vi "Initialize Transfer Groups.vi"(7 "FIFO Options":T1, 8 "error in (no error)":errorcluster, 10 "Transfer Group configurations":T2[](array[typedef]) {"Transfers"."channel blocks"."string descriptor"."buffer offset" format="%d bytes"; "Transfers"."channel blocks"."engine descriptor"."buffer offset" format="%d bytes"}, 11 "Plugin in":refnum<class "Plugin.lvclass">) -> (0 "error out":errorcluster, 2 "Transfer Groups":refnum<class "Transfer Group.lvclass">[](array[class]), 3 "Plugin out":refnum<class "Plugin.lvclass">)   [LabVIEW 2017, in "DSF Core.lvlib" / "Plugin.lvclass"]
uses:
  Plugin.lvclass
  DSF Configuration API/Public/Controls/DSF Engine Transfer Group Configuration.ctl
  DSF Configuration API/Public/Controls/DSF Direction.ctl
  DSF Configuration API/Public/Controls/DSF Timing Info.ctl
  DSF Configuration API/Public/Controls/DSF Settings Info.ctl
  DSF Configuration API/Public/Controls/DSF Engine Transfer Configuration.ctl
  DSF Configuration API/Public/Controls/DSF Byte Order.ctl
  DSF Configuration API/Public/Controls/DSF Engine Channel Configuration.ctl
  DSF Configuration API/Public/Controls/DSF Channel Buffer Descriptor.ctl
  DSF Configuration API/Public/Controls/DSF Data Type.ctl
  Transfer Group/Transfer Group.lvclass
  Typedefs/FIFO Flags.ctl
  Plugin.lvclass/Plugin.ctl
  Transfer Group/Transfer Group.lvclass/Transfer Group.ctl
  Shared/VIs/Sizeof.vi
  DSF Configuration API/Public/Required Buffer Size (Transfer Group).vi
  DSF Configuration API/Public/Channel Count (Transfer Group).vi
  DSF Core.lvlib
  Buffer/Buffers.lvclass
  Timing/Timing.lvclass
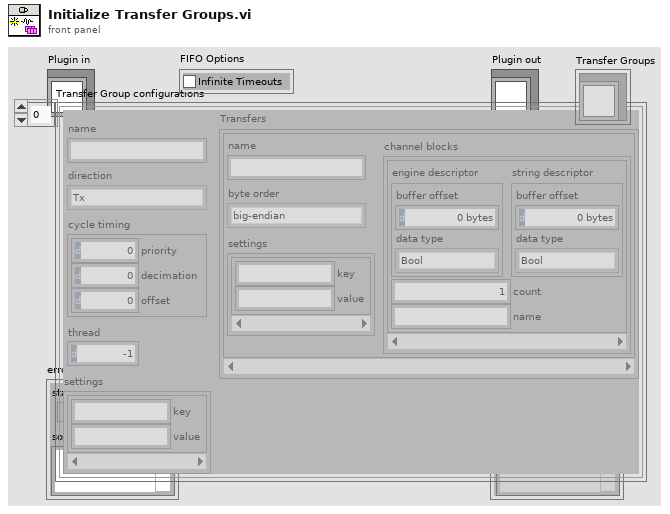
[diagram p1: front panel]
types:
  T1 = typedef "DSF Core.lvlib/FIFO Flags.ctl" = cluster{"Infinite Timeouts":bool}
  T2 = typedef "DSF Core.lvlib/DSF Engine Transfer Group Configuration.ctl" = cluster{"name":string, "direction":T3, "cycle timing":T4, "thread":i32, "settings":T5, "Transfers":T6[]}
  T3 = typedef "DSF Core.lvlib/DSF Direction.ctl" = enum8{"Tx", "Rx"}
  T4 = typedef "DSF Core.lvlib/DSF Timing Info.ctl" = cluster{"priority":u64, "decimation":u64, "offset":u64}
  T5 = typedef "DSF Core.lvlib/DSF Settings Info.ctl" = cluster{"key":string, "value":string}[]
  T6 = typedef "DSF Core.lvlib/DSF Engine Transfer Configuration.ctl" = cluster{"name":string, "byte order":T7, "channel blocks":T8[], "settings":T5}
  T7 = typedef "DSF Core.lvlib/DSF Byte Order.ctl" = enum8{"big-endian", "little-endian"}
  T8 = typedef "DSF Core.lvlib/DSF Engine Channel Configuration.ctl" = cluster{"engine descriptor":T9, "string descriptor":T9, "count":u64, "name":string}
  T9 = typedef "DSF Core.lvlib/DSF Channel Buffer Descriptor.ctl" = cluster{"buffer offset":u64, "data type":T10}
  T10 = typedef "DSF Core.lvlib/DSF Data Type.ctl" = enum8{"Bool", "SGL", "DBL", "I8", "I16", "I32", "I64", "U8", "U16", "U32", "U64"}
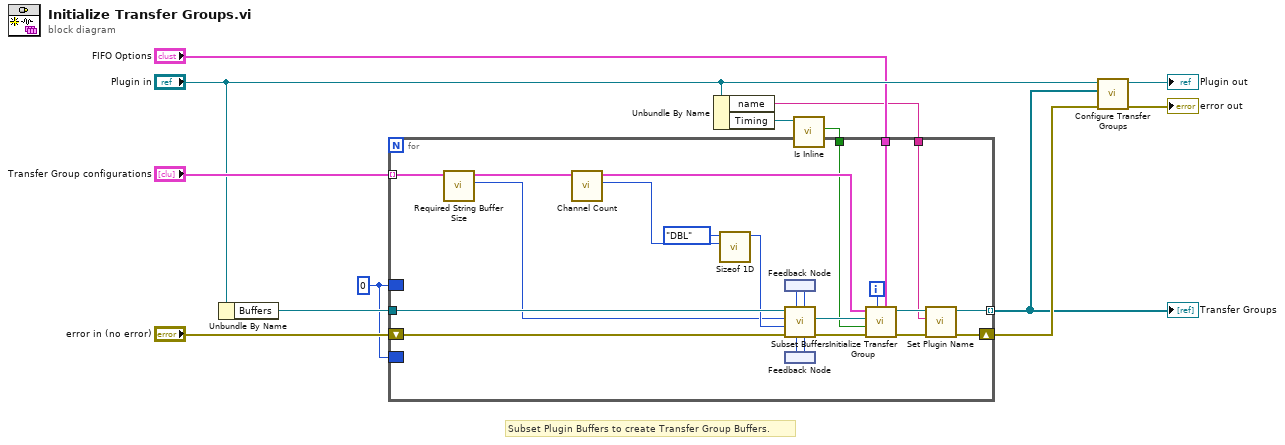
[diagram p0: block diagram]
diagram:
  w11 = u64 0 ("string buffer offset")
  # "Subset Plugin Buffers to create Transfer Group Buffers."
  n1 = Unbundle By Name("Plugin in") -> ("Buffers"=w13:refnum<class "Buffers.lvclass">)
  n2 = Unbundle By Name("Plugin in") -> ("name"=w1:string, "Timing"=w4:refnum<class "Timing.lvclass">)
  n3 = call "Is Inline.vi"("Timing in"=w4) -> ("inline?"=w6:bool)  [unwired: 9 in, 1 out]
  n4 = for {
    shift-right: [w35] -> w7
    shift-left: "error in (no error)" -> [w28]
    tunnel: [w15] -> w5 mode=indexing
    tunnel: w13 -> [w27]
    border: w11 -> [_]
    border: w11 -> [_]
    tunnel: "Transfer Group configurations" -> [w32] mode=indexing
    tunnel: w6 -> [w18]
    tunnel: "FIFO Options" -> [w17]
    tunnel: w1 -> [w14]
    i -> [w34]
    n5 = call-poly "Required String Buffer Size.vi"("Transfer Group Configuration in"=w32) -> ("required string buffer size"=w20:u64, "Transfer Group Configuration out"=w33:T2)  [unwired: 8 in, 1 out]
    n6 = call-poly "Channel Count.vi"("Transfer Group Configuration in"=w33) -> ("total channel count"=w29:u64, "Transfer Group Configuration out"=w31:T2)  [unwired: 8 in, 1 out]
    n7 = call "Sizeof 1D.vi"("count"=w29, "data type"=DSF_Data_Type."DBL") -> ("size in bytes"=w21:u64)  [unwired: 9 in]
    n8 = feedback #1() -> (w22:u64)
    n9 = feedback #2() -> (w24:u64)
    n10 = call "Subset Buffers.vi"("inline buffer offset"=w24, "string buffer offset"=w22, "error in (no error)"=w28, "inline buffer size"=w21, "string buffer size"=w20, "Buffers in"=w27) -> ("error out"=w26:errorcluster, "subset Buffers"=w19:refnum<class "Buffers.lvclass">, "inline buffer offset +size"=w25:u64, "string buffer offset + size"=w23:u64)  [unwired: 1 in, 1 out]
    n11 = feedback-in #1(w23) -> ()
    n12 = feedback-in #2(w25) -> ()
    n13 = call "Initialize Transfer Group.vi"("FIFO Options"=w17, "id"=w34, "error in (no error)"=w26, "force inline? (F)"=w18, "Transfer Group Buffers"=w19, "Transfer Group Configuration"=w31) -> ("error out"=w35:errorcluster, "Transfer Group out"=w16:refnum<class "Transfer Group.lvclass">)  [unwired: 4 in]
    n14 = call "Set Plugin Name.vi"("plugin"=w14, "Transfer Group in"=w16) -> ("Transfer Group out"=w15:refnum<class "Transfer Group.lvclass">)  [unwired: 9 in]
  }
  "Transfer Groups" <- w5
  n15 = call "Configure Transfer Groups.vi"("error in (no error)"=w7, "Transfer Groups"=w5, "Plugin in"="Plugin in") -> ("error out"=→"error out":errorcluster, "Plugin out"=→"Plugin out":refnum<class "Plugin.lvclass">)  [unwired: 7 in]
